vi "Simplified WB Spectrum Sense.vi"() -> ()   [LabVIEW 2015]
panel:
  in  "Rx Parameters":T1={"IQ Sampling\nRate [S/sec]"=200000.0, "Acq Duration [sec]"=0.002, "LO Frequency"=88000000.0, "Bandwidth"=108000000.0, "Gain [dB]"=29.0, "Active Antenna"="RX1", "Reference Source"="Internal", "Timebase Source"="Internal"} {"Gain [dB]" format="%#_4g"; "Bandwidth" min=50000000.0 max=6000000000.0 step=1000.0 format="%#.15p"; "LO Frequency" min=50000000.0 max=6000000000.0 step=1000.0 format="%#.15p"; "Acq Duration [sec]" min=0.0 step=0.001 format="%#.6p"; "IQ Sampling\nRate [S/sec]" format="%#_6p"}
  in  "Display Settings":cluster{"display unit":u16, "log/linear":u16}={"display unit"=2, "log/linear"=2} {"log/linear" items=["Linear", "dB", "dBm"]; "display unit" items=["Vrms", "Vpk", "Vrms^2", "Vpk^2", "Vrms/rtHz", "Vpk/rtHz", "Vrms^2/Hz", "Vpk^2/Hz"]}
  out "error out":errorcluster
  out "FFT Power Spectrum":cluster{"f0":dbl, "df":dbl, "IQ":dbl[]}(graph)={"f0"=87950000.0, "df"=500.0, "IQ"=array[40200 elements]}
  in  "USRP IP Address":refnum<k15>="192.168.10.3"
  # "Wideband Spectrum"
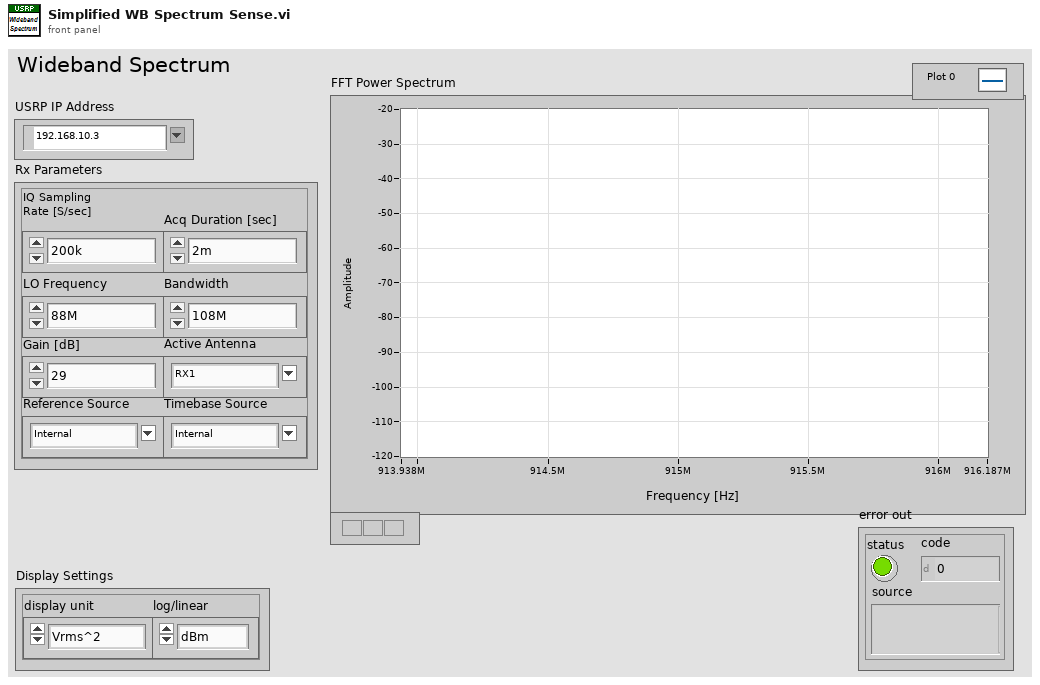
[diagram p1: front panel]
types:
  T1 = cluster{"IQ Sampling\nRate [S/sec]":dbl, "Acq Duration [sec]":dbl, "LO Frequency":dbl, "Bandwidth":dbl, "Gain [dB]":dbl, "Active Antenna":string, "Reference Source":string, "Timebase Source":string}
  T2 = typedef "subFrameParams.ctl" = cluster{"IQ Rate":dbl, "Frames":i32, "Length of Subset":i32, "Start Index of Subset":i32, "Start Carrier [Hz]":dbl, "Stop Carrier [Hz]":dbl, "Acq Duration [sec]":dbl}
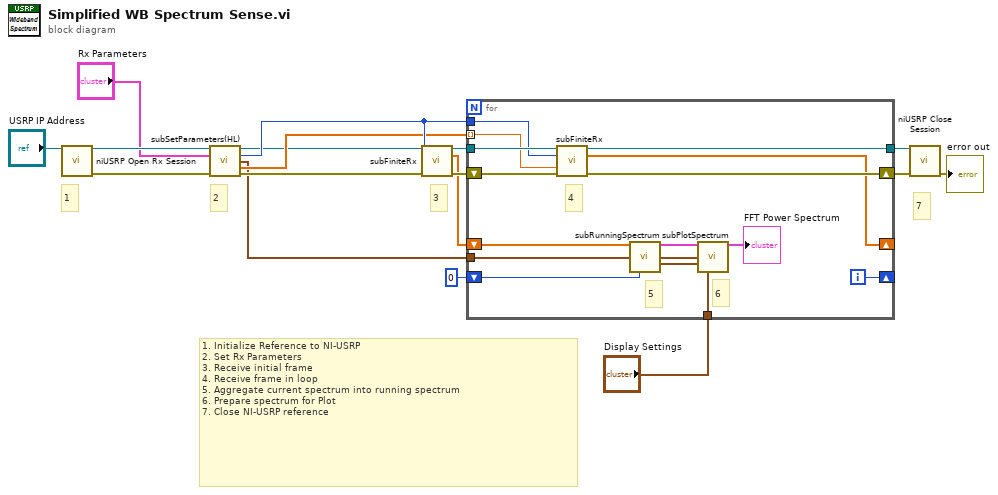
[diagram p0: block diagram]
diagram:
  # "7"
  # "3"
  # "2"
  # "1"
  # "1. Initialize Reference to NI-USRP\n2. Set Rx Parameters\n3. Receive initial frame\n4. Receive frame in loop\n5. Aggregate current spectrum into running spectrum\n6. Prepare spectrum for Plot\n7. Close NI-USRP reference"
  n1 = call <instrlib>:"niUSRP Open Rx Session.vi"("device names"="USRP IP Address") -> ("session handle out"=w10:refnum<k15>, "error out"=w9:errorcluster)  [unwired: 13 in]
  n2 = call "subSetParameters(HL).vi"("IVI Refnum in"=w10, "Rx Parameters"="Rx Parameters", "error in (no error)"=w9) -> ("IVI Refnum out"=w3:refnum<k15>, "samples per acquisition"=w12:i32, "Frame Parameters"=w1:T2, "test carrier frequencies"=w7:dbl[], "error out"=w2:errorcluster)  [unwired: 8 in]
  n3 = call "subFiniteRx.vi"("IVI Refnum in"=w3, "Number of Samples"=w12, "error in (no error)"=w2) -> ("IVI Refnum out"=w13:refnum<k15>, "data"=w5:cdb[], "error out"=w14:errorcluster)  [unwired: 10 in]
  n4 = for {
    tunnel: w13 -> [w33]
    tunnel: w12 -> [w21]
    tunnel: [w32] -> w16
    shift-right: [w31] -> w15
    shift-left: w14 -> [w30]
    shift-right: [w22] -> _
    shift-left: w5 -> [w29]
    tunnel: w7 -> [w26] mode=indexing
    tunnel: "Display Settings" -> [w23]
    shift-right: [w20] -> _
    shift-left: 0 -> [w19]
    tunnel: w1 -> [w18]
    i -> [w20]
    # "6"
    # "5"
    # "4"
    n5 = call "subFiniteRx.vi"("IVI Refnum in"=w33, "Number of Samples"=w21, "Carrier Frequency"=w26, "error in (no error)"=w30) -> ("IVI Refnum out"=w32:refnum<k15>, "data"=w22:cdb[], "error out"=w31:errorcluster)  [unwired: 9 in]
    n6 = call "subRunningSpectrum.vi"("Input Baseband IQ"=w29, "Frame Parameters"=w18, "Iteration"=w19) -> ("Spectrum to Plot"=w28:cluster{"f0":dbl, "df":dbl, "IQ":dbl[]}, "Frame Parameters out"=w25:T2, "window properties"=w24:cluster{"eq noise BW":dbl, "coherent gain":dbl})  [unwired: 9 in, 1 out]
    n7 = call "subPlotSpectrum.vi"("Spectrum to Plot"=w28, "Frame Parameters"=w25, "window properties"=w24, "Display"=w23) -> ("Spectrum to Plot"=→"FFT Power Spectrum":cluster{"f0":dbl, "df":dbl, "IQ":dbl[]})  [unwired: 11 in]
  }
  n8 = call <instrlib>:"niUSRP Close Session.vi"("session handle"=w16, "error in (no error)"=w15) -> ("error out"=→"error out":errorcluster)  [unwired: 13 in]
